vi "WaitForEdge.better.fpga.vi"(8 "Timeout":i32, 10 "Sync":u16) -> ()   [LabVIEW 2012]
uses:
  <vilib>/rvi/eio/common/nirviEmuTemplateMethod_errors.vi
  <vilib>/eio/EIOMethodNode/EIOMethodNode.xnode
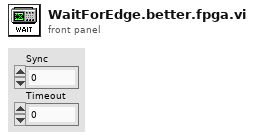
[diagram p1: front panel]
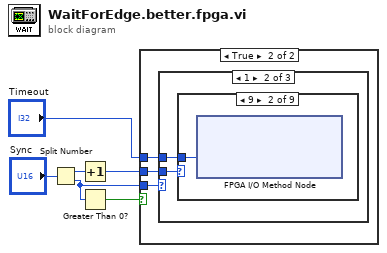
[diagram p0: block diagram]
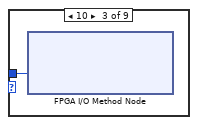
[diagram p5: hidden frame]
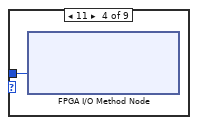
[diagram p6: hidden frame]
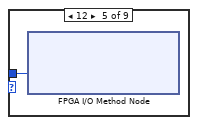
[diagram p7: hidden frame]
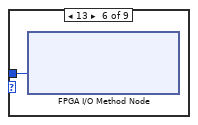
[diagram p8: hidden frame]
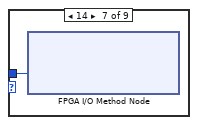
[diagram p9: hidden frame]
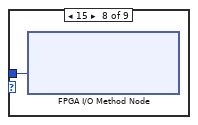
[diagram p10: hidden frame]
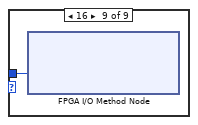
[diagram p11: hidden frame]
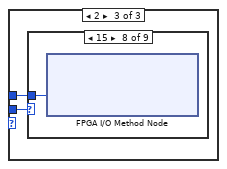
[diagram p12: hidden frame]
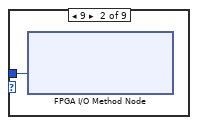
[diagram p14: hidden frame]
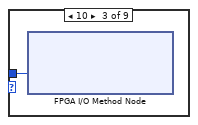
[diagram p15: hidden frame]
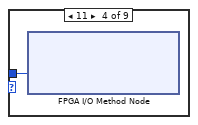
[diagram p16: hidden frame]
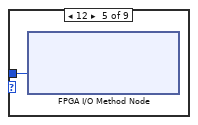
[diagram p17: hidden frame]
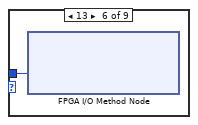
[diagram p18: hidden frame]
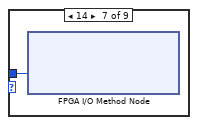
[diagram p19: hidden frame]
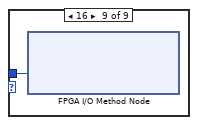
[diagram p20: hidden frame]
diagram:
  n1 = Split Number(x="Sync") -> (hi(x)=w3:u8, lo(x)=w4:u8)
  n2 = Increment(x=w3) -> (x+1=w2:u8)
  n3 = Greater Than 0?(x=w4) -> (x > 0?=w5:bool)
  n4 = case shown="True" w5 {
    tunnel: w2 -> [_ w9]
    tunnel: w4 -> [_ w8]
    tunnel: "Timeout" -> [_ w7]
    frame False {
    }
    frame True {
      n5 = case shown="1" w8 {
        tunnel: w9 -> [_ w11 w21]
        tunnel: w7 -> [_ w10 w20]
        frame 0, Default {
        }
        frame 1 {
          n6 = case shown="9" w11 {
            tunnel: w10 -> [_ w12 w13 w14 w15 w16 w17 w18 w19]
            frame 0, Default {
            }
            frame 9 {
              n7 = xnode "FPGA I/O Method Node"("Timeout"=w12) -> ()  [unwired: 1 in, 2 out]
            }
            frame 10 {
              n8 = xnode "FPGA I/O Method Node"("Timeout"=w13) -> ()  [unwired: 1 in, 2 out]
            }
            frame 11 {
              n9 = xnode "FPGA I/O Method Node"("Timeout"=w14) -> ()  [unwired: 1 in, 2 out]
            }
            frame 12 {
              n10 = xnode "FPGA I/O Method Node"("Timeout"=w15) -> ()  [unwired: 1 in, 2 out]
            }
            frame 13 {
              n11 = xnode "FPGA I/O Method Node"("Timeout"=w16) -> ()  [unwired: 1 in, 2 out]
            }
            frame 14 {
              n12 = xnode "FPGA I/O Method Node"("Timeout"=w17) -> ()  [unwired: 1 in, 2 out]
            }
            frame 15 {
              n13 = xnode "FPGA I/O Method Node"("Timeout"=w18) -> ()  [unwired: 1 in, 2 out]
            }
            frame 16 {
              n14 = xnode "FPGA I/O Method Node"("Timeout"=w19) -> ()  [unwired: 1 in, 2 out]
            }
          }
        }
        frame 2 {
          n15 = case shown="15" w21 {
            tunnel: w20 -> [_ w22 w23 w24 w25 w26 w27 w28 w29]
            frame 0, Default {
            }
            frame 9 {
              n16 = xnode "FPGA I/O Method Node"("Timeout"=w22) -> ()  [unwired: 1 in, 2 out]
            }
            frame 10 {
              n17 = xnode "FPGA I/O Method Node"("Timeout"=w23) -> ()  [unwired: 1 in, 2 out]
            }
            frame 11 {
              n18 = xnode "FPGA I/O Method Node"("Timeout"=w24) -> ()  [unwired: 1 in, 2 out]
            }
            frame 12 {
              n19 = xnode "FPGA I/O Method Node"("Timeout"=w25) -> ()  [unwired: 1 in, 2 out]
            }
            frame 13 {
              n20 = xnode "FPGA I/O Method Node"("Timeout"=w26) -> ()  [unwired: 1 in, 2 out]
            }
            frame 14 {
              n21 = xnode "FPGA I/O Method Node"("Timeout"=w27) -> ()  [unwired: 1 in, 2 out]
            }
            frame 15 {
              n22 = xnode "FPGA I/O Method Node"("Timeout"=w28) -> ()  [unwired: 1 in, 2 out]
            }
            frame 16 {
              n23 = xnode "FPGA I/O Method Node"("Timeout"=w29) -> ()  [unwired: 1 in, 2 out]
            }
          }
        }
      }
    }
  }
